vi "Check Motor Fault bit.vi"(5 "Status Byte":u16 format="%x") -> (6 "Motor Fault?":bool)   [LabVIEW 2015, in "Tool Module.lvlib"]
uses:
  Tool Module.lvlib
  _Status Bits Typedef.ctl
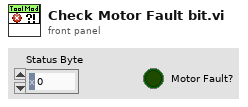
[diagram p1: front panel]
types:
  T1 = typedef "Tool Module.lvlib/_Status Bits Typedef.ctl" = u16
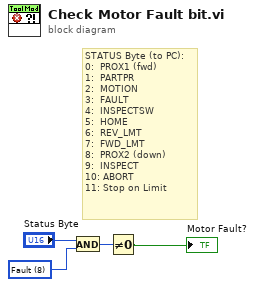
[diagram p0: block diagram]
diagram:
  w1 = T1 8 items=["PROX1"=1, "PartPresent"=2, "Motion"=4, "Fault"=8, "Switch"=16, "Home"=32, "RLS"=64, "FLS"=128, "PROX2"=256, "INSPECT"=512, "Abort"=1024, "Stop on Limit"=2048] ("_Status bit values typedef")
  # "STATUS Byte (to PC):\n0:  PROX1 (fwd)\n1:  PARTPR\n2:  MOTION\n3:  FAULT\n4:  INSPECTSW\n5:  HOME\n6:  REV_LMT\n7:  FWD_LMT\n8:  PROX2 (down)\n9:  INSPECT\n10: ABORT\n11: Stop on Limit"
  n1 = And(x="Status Byte", y=w1) -> (x .and. y?=w3:T1)
  n2 = Not Equal To 0?(x=w3) -> (x != 0?=→"Motor Fault?":bool)
